vi "get_TIFF_description.vi"(8 "error in (no error)":errorcluster, 10 "page":i32, 11 "path in":path) -> (0 "error out":errorcluster, 2 "description":string, 3 "path out":path, 4 "description empty?":bool)   [LabVIEW 2010, in "TIFFManagement.lvlib"]
uses:
  TIFFManagement.lvlib
  VisualCPP/Release/TIFFManagement.dll
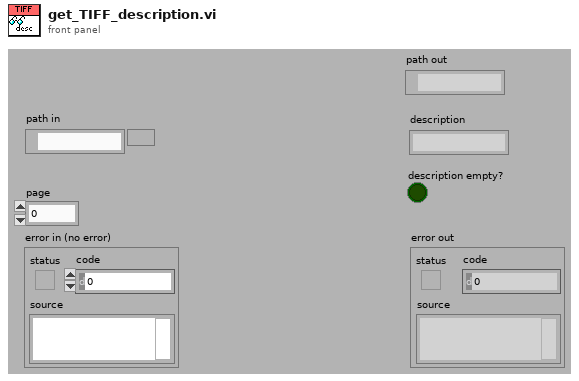
[diagram p1: front panel]
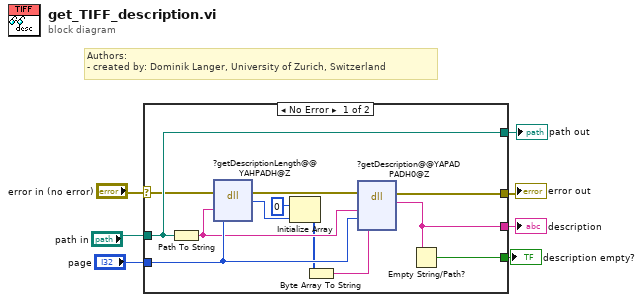
[diagram p0: block diagram]
diagram:
  # "Authors: \n- created by: Dominik Langer, University of Zurich, Switzerland"
  n1 = case shown="No Error" "error in (no error)" {
    selector: "error in (no error)" -> [w15 w21]
    tunnel: [w19 w21] -> w6
    tunnel: "page" -> [w13 _]
    tunnel: "path in" -> [w18 w20]
    tunnel: [w18 w20] -> w3
    tunnel: [w17 _] -> w2
    tunnel: [w16 _] -> w1
    frame No Error {
      n2 = Path To String(path=w18) -> (string=w12:string)
      n3 = dll-call lib="C:/helioscan/common/libraries/TIFFManagement/VisualCPP/Release/TIFFManagement.dll" fn="?getDescriptionLength@@YAHPADH@Z" label="TIFFManagement.dll:getDescriptionLength"(error in=w15, "path"=w12, "page"=w13) -> (error out=w14:errorcluster, "return type"=w11:i32)  [unwired: 4 in, 1 out]
      n4 = Initialize Array(u8 0, w11) -> (w9:u8[])
      n5 = Byte Array To String(unsigned byte array=w9) -> (string=w8:string)
      n6 = dll-call lib="C:/helioscan/common/libraries/TIFFManagement/VisualCPP/Release/TIFFManagement.dll" fn="?getDescription@@YAPADPADH0@Z" label="TIFFManagement.dll:getDescription"(error in=w14, "path"=w12, "page"=w13, "description"=w8) -> (error out=w19:errorcluster, "return type"=w16:string)  [unwired: 5 in, 1 out]
      n7 = Empty String/Path?(string/path=w16) -> (empty?=w17:bool)
    }
    frame Error {
    }
  }
  "description" <- w1
  "error out" <- w6
  "path out" <- w3
  "description empty?" <- w2
